vi "WILT Step 1.vi"(7 "Station Number":u32, 8 "Error In":errorcluster, 10 "Station Test State Cluster":T5, 11 "Dryer Control Input":T1 {"Night Cycle Count" format="%04d"; "Day Cycle Count" format="%04d"}) -> (0 "Error Out":errorcluster, 2 "Step 1 Output":T5, 3 "Step 1 Output":T1 {"Night Cycle Count" format="%04d"; "Day Cycle Count" format="%04d"})   [LabVIEW 2016]
uses:
  Type Definitions/WILT Dryer.ctl
  Type Definitions/WILT Dryer Details.ctl
  Type Definitions/WILT Agilent Channel Definition.ctl
  Type Definitions/WILT DAQ Data.ctl
  Type Definitions/WILT Station Test State Cluster.ctl
  Type Definitions/WILT Dryer Test State.ctl
  Globals/WILT Globals Main Program.vi
panel:
  # "Day"
  # "Night"
  # "Day"
  # "Night"
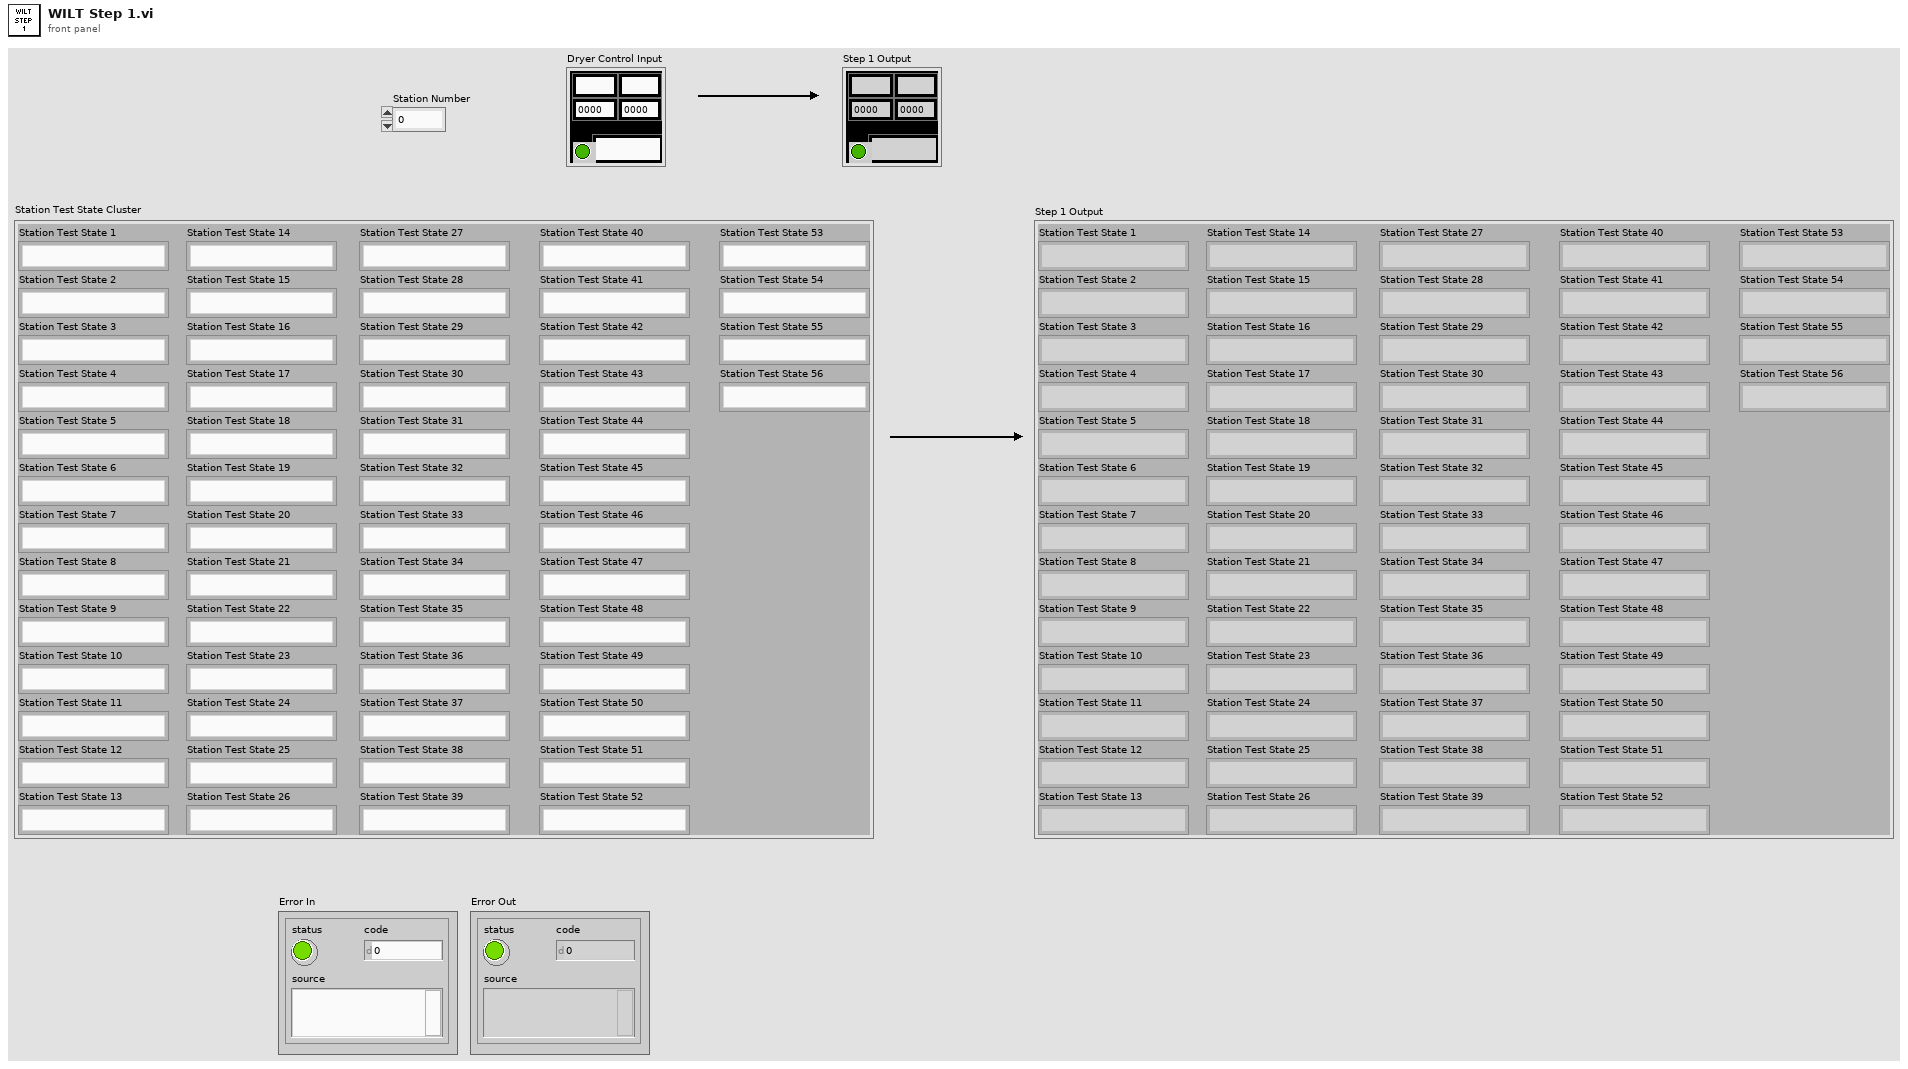
[diagram p1: front panel]
types:
  T1 = typedef "WILT Dryer.ctl" = cluster{"Lab ID":string, "Day Cycle Count":i32, "Station Label":string, "Dryer Details":T2, "Status Color":u32, "Invisible Button":bool, "Night Cycle Count":i32, "Station Index":i32, "Cycle Index":string, "Audit Alert":bool, "Agilent Channel Definition":T3, "DAQ Data":T4}
  T2 = typedef "WILT Dryer Details.ctl" = cluster{"Station":string, "Lab ID":string, "TR Number":string}
  T3 = typedef "WILT Agilent Channel Definition.ctl" = cluster{"Channel":string, "Station":string, "Label":string, "Agilent Station":string, "Data":dbl}
  T4 = typedef "WILT DAQ Data.ctl" = cluster{"L1 Current":dbl, "L2 Current":dbl, "Temperature  Deg F (TC)":dbl, "Volts":dbl, "Volts (208)":dbl, "SW (208)":dbl}
  T5 = typedef "WILT Station Test State Cluster.ctl" = cluster{"Station Test State 1":T6, "Station Test State 2":T6, "Station Test State 3":T6, "Station Test State 4":T6, "Station Test State 5":T6, "Station Test State 6":T6, "Station Test State 7":T6, "Station Test State 8":T6, "Station Test State 9":T6, "Station Test State 10":T6, "Station Test State 11":T6, "Station Test State 12":T6, "Station Test State 13":T6, "Station Test State 14":T6, "Station Test State 15":T6, "Station Test State 16":T6, "Station Test State 17":T6, "Station Test State 18":T6, "Station Test State 19":T6, "Station Test State 20":T6, "Station Test State 21":T6, "Station Test State 22":T6, "Station Test State 23":T6, "Station Test State 24":T6, "Station Test State 25":T6, "Station Test State 26":T6, "Station Test State 27":T6, "Station Test State 28":T6, "Station Test State 29":T6, "Station Test State 30":T6, "Station Test State 31":T6, "Station Test State 32":T6, "Station Test State 33":T6, "Station Test State 34":T6, "Station Test State 35":T6, "Station Test State 36":T6, "Station Test State 37":T6, "Station Test State 38":T6, "Station Test State 39":T6, "Station Test State 40":T6, "Station Test State 41":T6, "Station Test State 42":T6, "Station Test State 43":T6, "Station Test State 44":T6, "Station Test State 45":T6, "Station Test State 46":T6, "Station Test State 47":T6, "Station Test State 48":T6, "Station Test State 49":T6, "Station Test State 50":T6, "Station Test State 51":T6, "Station Test State 52":T6, "Station Test State 53":T6, "Station Test State 54":T6, "Station Test State 55":T6, "Station Test State 56":T6}
  T6 = typedef "WILT Dryer Test State.ctl" = enum16{"No Serial Number", "Waiting for Dryer To Start", "Drying Clothes", "Water Injection 1 (On)", "Water Injection 1 Timer", "Water Injection 1 (Off)", "Pause Dryer", "Sending Start Stop CMD", "Pause Dryer 2", "Sending Start Stop CMD 2", "Drying Clothes 2", "Water Injection 2 (On)", "Water Injection 2 Timer", "Water Injection 2 (Off)", "Drying Clothes 3", "Cooling Down", "Sending Start Stop CMD 3", "Increment Cycle"}
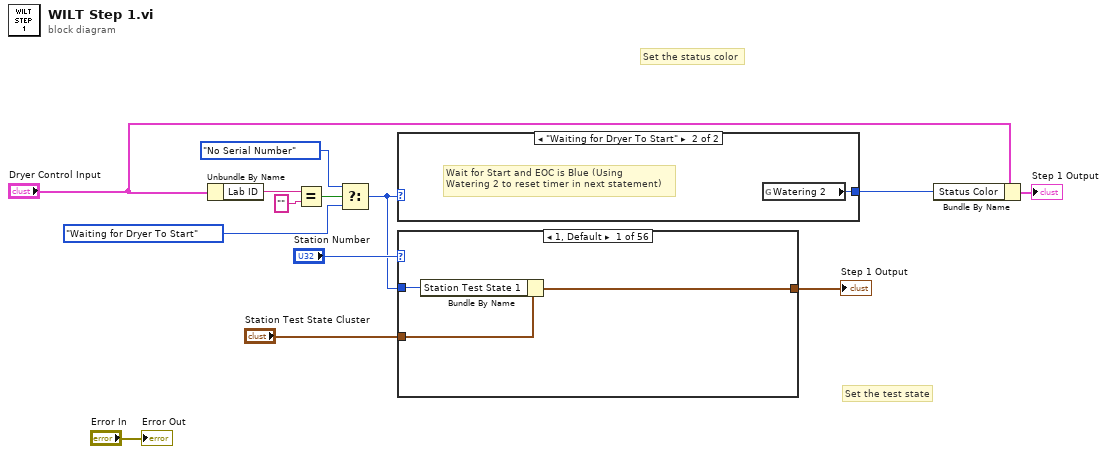
[diagram p0: block diagram]
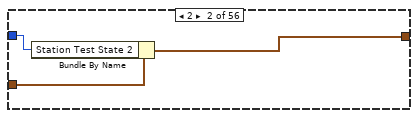
[diagram p2: hidden frame]
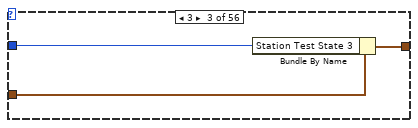
[diagram p3: hidden frame]
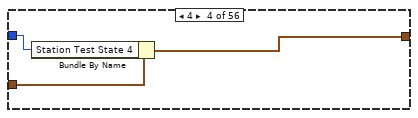
[diagram p4: hidden frame]
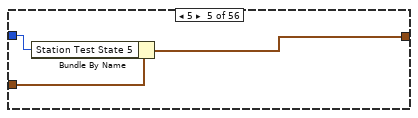
[diagram p5: hidden frame]
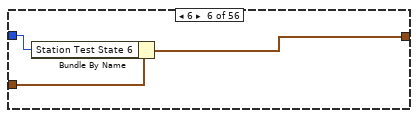
[diagram p6: hidden frame]
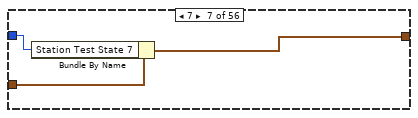
[diagram p7: hidden frame]
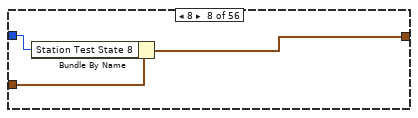
[diagram p8: hidden frame]
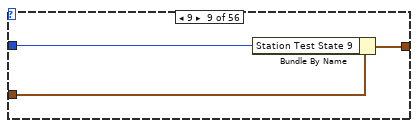
[diagram p9: hidden frame]
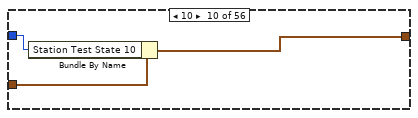
[diagram p10: hidden frame]
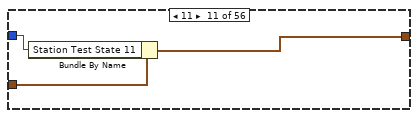
[diagram p11: hidden frame]
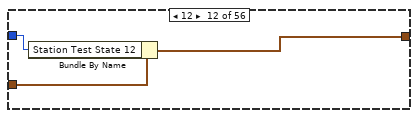
[diagram p12: hidden frame]
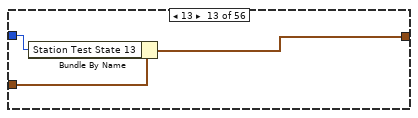
[diagram p13: hidden frame]
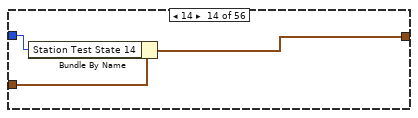
[diagram p14: hidden frame]
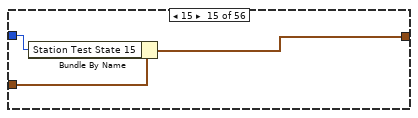
[diagram p15: hidden frame]
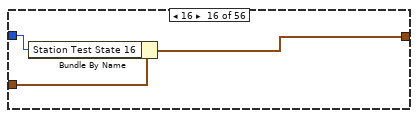
[diagram p16: hidden frame]
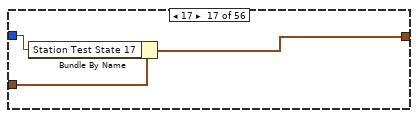
[diagram p17: hidden frame]
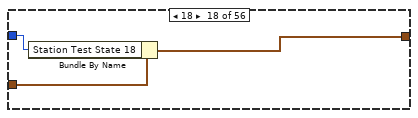
[diagram p18: hidden frame]
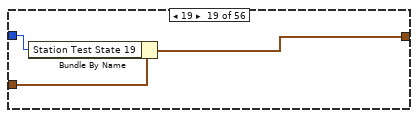
[diagram p19: hidden frame]
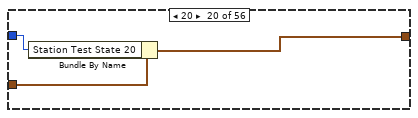
[diagram p20: hidden frame]
diagram:
  # "Set the status color"
  # "Set the test state"
  n1 = Unbundle By Name("Dryer Control Input") -> ("Lab ID"=w9:string)
  n2 = Equal?(x=w9, y="") -> (x = y?=w11:bool)
  n3 = Select(t=WILT_Dryer_Test_State."No Serial Number" ("Test State"), s=w11, f=WILT_Dryer_Test_State."Waiting for Dryer To Start" ("Test State")) -> (s? t:f=w4:T6)
  n4 = case shown="\"Waiting for Dryer To Start\"" w4 {
    tunnel: [w14 w15] -> w7
    frame "No Serial Number", Default {
      n5 = global read "WILT Globals Main Program.vi" "Color Uncofigured"() -> (w14:u32)
    }
    frame "Waiting for Dryer To Start" {
      # "Wait for Start and EOC is Blue (Using\nWatering 2 to reset timer in next statement)"
      n6 = global read "WILT Globals Main Program.vi" "Watering 2"() -> (w15:u32)
    }
  }
  n7 = case shown="1, Default" "Station Number" {
    tunnel: "Station Test State Cluster" -> [w18 w21 w24 w27 w30 w33 w36 w39 w42 w45 w48 w51 w54 w57 w60 w63 w66 w69 w72 w75 w78 w81 w84 w87 w90 w93 w96 w99 w102 w105 w108 w111 w114 w117 w120 w123 w126 w129 w132 w135 w138 w141 w144 w147 w150 w153 w156 w159 w162 w165 w168 w171 w174 w177 w180 w183]
    tunnel: w4 -> [w17 w19 w22 w25 w28 w31 w34 w37 w40 w43 w46 w49 w52 w55 w58 w61 w64 w67 w70 w73 w76 w79 w82 w85 w88 w91 w94 w97 w100 w103 w106 w109 w112 w115 w118 w121 w124 w127 w130 w133 w136 w139 w142 w145 w148 w151 w154 w157 w160 w163 w166 w169 w172 w175 w178 w181]
    tunnel: [w16 w20 w23 w26 w29 w32 w35 w38 w41 w44 w47 w50 w53 w56 w59 w62 w65 w68 w71 w74 w77 w80 w83 w86 w89 w92 w95 w98 w101 w104 w107 w110 w113 w116 w119 w122 w125 w128 w131 w134 w137 w140 w143 w146 w149 w152 w155 w158 w161 w164 w167 w170 w173 w176 w179 w182] -> w3
    frame 1, Default {
      n8 = Bundle By Name(cluster=w18, "Station Test State 1"=w17) -> (w16:T5)
    }
    frame 2 {
      n9 = Bundle By Name(cluster=w21, "Station Test State 2"=w19) -> (w20:T5)
    }
    frame 3 {
      n10 = Bundle By Name(cluster=w24, "Station Test State 3"=w22) -> (w23:T5)
    }
    frame 4 {
      n11 = Bundle By Name(cluster=w27, "Station Test State 4"=w25) -> (w26:T5)
    }
    frame 5 {
      n12 = Bundle By Name(cluster=w30, "Station Test State 5"=w28) -> (w29:T5)
    }
    frame 6 {
      n13 = Bundle By Name(cluster=w33, "Station Test State 6"=w31) -> (w32:T5)
    }
    frame 7 {
      n14 = Bundle By Name(cluster=w36, "Station Test State 7"=w34) -> (w35:T5)
    }
    frame 8 {
      n15 = Bundle By Name(cluster=w39, "Station Test State 8"=w37) -> (w38:T5)
    }
    frame 9 {
      n16 = Bundle By Name(cluster=w42, "Station Test State 9"=w40) -> (w41:T5)
    }
    frame 10 {
      n17 = Bundle By Name(cluster=w45, "Station Test State 10"=w43) -> (w44:T5)
    }
    frame 11 {
      n18 = Bundle By Name(cluster=w48, "Station Test State 11"=w46) -> (w47:T5)
    }
    frame 12 {
      n19 = Bundle By Name(cluster=w51, "Station Test State 12"=w49) -> (w50:T5)
    }
    frame 13 {
      n20 = Bundle By Name(cluster=w54, "Station Test State 13"=w52) -> (w53:T5)
    }
    frame 14 {
      n21 = Bundle By Name(cluster=w57, "Station Test State 14"=w55) -> (w56:T5)
    }
    frame 15 {
      n22 = Bundle By Name(cluster=w60, "Station Test State 15"=w58) -> (w59:T5)
    }
    frame 16 {
      n23 = Bundle By Name(cluster=w63, "Station Test State 16"=w61) -> (w62:T5)
    }
    frame 17 {
      n24 = Bundle By Name(cluster=w66, "Station Test State 17"=w64) -> (w65:T5)
    }
    frame 18 {
      n25 = Bundle By Name(cluster=w69, "Station Test State 18"=w67) -> (w68:T5)
    }
    frame 19 {
      n26 = Bundle By Name(cluster=w72, "Station Test State 19"=w70) -> (w71:T5)
    }
    frame 20 {
      n27 = Bundle By Name(cluster=w75, "Station Test State 20"=w73) -> (w74:T5)
    }
    frame 21 {
      n28 = Bundle By Name(cluster=w78, "Station Test State 21"=w76) -> (w77:T5)
    }
    frame 22 {
      n29 = Bundle By Name(cluster=w81, "Station Test State 22"=w79) -> (w80:T5)
    }
    frame 23 {
      n30 = Bundle By Name(cluster=w84, "Station Test State 23"=w82) -> (w83:T5)
    }
    frame 24 {
      n31 = Bundle By Name(cluster=w87, "Station Test State 24"=w85) -> (w86:T5)
    }
    frame 25 {
      n32 = Bundle By Name(cluster=w90, "Station Test State 25"=w88) -> (w89:T5)
    }
    frame 26 {
      n33 = Bundle By Name(cluster=w93, "Station Test State 26"=w91) -> (w92:T5)
    }
    frame 27 {
      n34 = Bundle By Name(cluster=w96, "Station Test State 27"=w94) -> (w95:T5)
    }
    frame 28 {
      n35 = Bundle By Name(cluster=w99, "Station Test State 28"=w97) -> (w98:T5)
    }
    frame 29 {
      n36 = Bundle By Name(cluster=w102, "Station Test State 29"=w100) -> (w101:T5)
    }
    frame 30 {
      n37 = Bundle By Name(cluster=w105, "Station Test State 30"=w103) -> (w104:T5)
    }
    frame 31 {
      n38 = Bundle By Name(cluster=w108, "Station Test State 31"=w106) -> (w107:T5)
    }
    frame 32 {
      n39 = Bundle By Name(cluster=w111, "Station Test State 32"=w109) -> (w110:T5)
    }
    frame 33 {
      n40 = Bundle By Name(cluster=w114, "Station Test State 33"=w112) -> (w113:T5)
    }
    frame 34 {
      n41 = Bundle By Name(cluster=w117, "Station Test State 34"=w115) -> (w116:T5)
    }
    frame 35 {
      n42 = Bundle By Name(cluster=w120, "Station Test State 35"=w118) -> (w119:T5)
    }
    frame 36 {
      n43 = Bundle By Name(cluster=w123, "Station Test State 36"=w121) -> (w122:T5)
    }
    frame 37 {
      n44 = Bundle By Name(cluster=w126, "Station Test State 37"=w124) -> (w125:T5)
    }
    frame 38 {
      n45 = Bundle By Name(cluster=w129, "Station Test State 38"=w127) -> (w128:T5)
    }
    frame 39 {
      n46 = Bundle By Name(cluster=w132, "Station Test State 39"=w130) -> (w131:T5)
    }
    frame 40 {
      n47 = Bundle By Name(cluster=w135, "Station Test State 40"=w133) -> (w134:T5)
    }
    frame 41 {
      n48 = Bundle By Name(cluster=w138, "Station Test State 41"=w136) -> (w137:T5)
    }
    frame 42 {
      n49 = Bundle By Name(cluster=w141, "Station Test State 42"=w139) -> (w140:T5)
    }
    frame 43 {
      n50 = Bundle By Name(cluster=w144, "Station Test State 43"=w142) -> (w143:T5)
    }
    frame 44 {
      n51 = Bundle By Name(cluster=w147, "Station Test State 44"=w145) -> (w146:T5)
    }
    frame 45 {
      n52 = Bundle By Name(cluster=w150, "Station Test State 45"=w148) -> (w149:T5)
    }
    frame 46 {
      n53 = Bundle By Name(cluster=w153, "Station Test State 46"=w151) -> (w152:T5)
    }
    frame 47 {
      n54 = Bundle By Name(cluster=w156, "Station Test State 47"=w154) -> (w155:T5)
    }
    frame 48 {
      n55 = Bundle By Name(cluster=w159, "Station Test State 48"=w157) -> (w158:T5)
    }
    frame 49 {
      n56 = Bundle By Name(cluster=w162, "Station Test State 49"=w160) -> (w161:T5)
    }
    frame 50 {
      n57 = Bundle By Name(cluster=w165, "Station Test State 50"=w163) -> (w164:T5)
    }
    frame 51 {
      n58 = Bundle By Name(cluster=w168, "Station Test State 51"=w166) -> (w167:T5)
    }
    frame 52 {
      n59 = Bundle By Name(cluster=w171, "Station Test State 52"=w169) -> (w170:T5)
    }
    frame 53 {
      n60 = Bundle By Name(cluster=w174, "Station Test State 53"=w172) -> (w173:T5)
    }
    frame 54 {
      n61 = Bundle By Name(cluster=w177, "Station Test State 54"=w175) -> (w176:T5)
    }
    frame 55 {
      n62 = Bundle By Name(cluster=w180, "Station Test State 55"=w178) -> (w179:T5)
    }
    frame 56 {
      n63 = Bundle By Name(cluster=w183, "Station Test State 56"=w181) -> (w182:T5)
    }
  }
  "Step 1 Output" <- w3
  n64 = Bundle By Name(cluster="Dryer Control Input", "Status Color"=w7) -> (→"Step 1 Output":T1)
  "Error Out" <- "Error In"
